vi "mrq_move.vi"(0 "ax":i32, 1 "VISA资源名称":refnum<visa-resource-name>, 2 "page":i32, 3 "t":sgl=1.0, 4 "endV":sgl, 5 "angle":sgl=360.0, 8 "错误输入（无错误）":errorcluster) -> (6 "VISA资源名称输出":refnum<visa-resource-name>, 7 "错误输出":errorcluster)   [LabVIEW 2017]
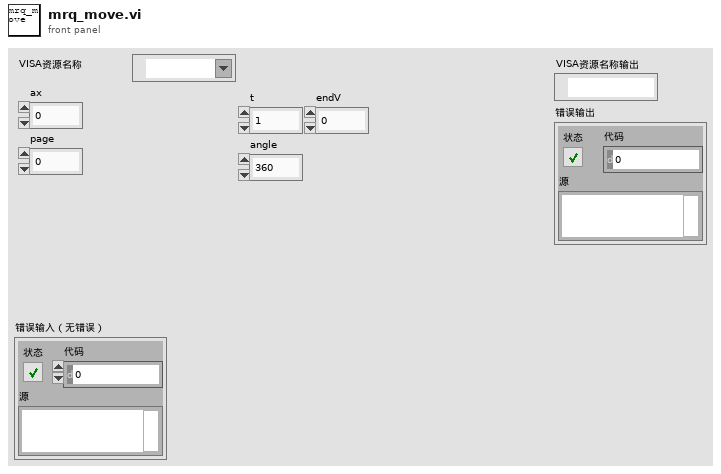
[diagram p1: front panel]
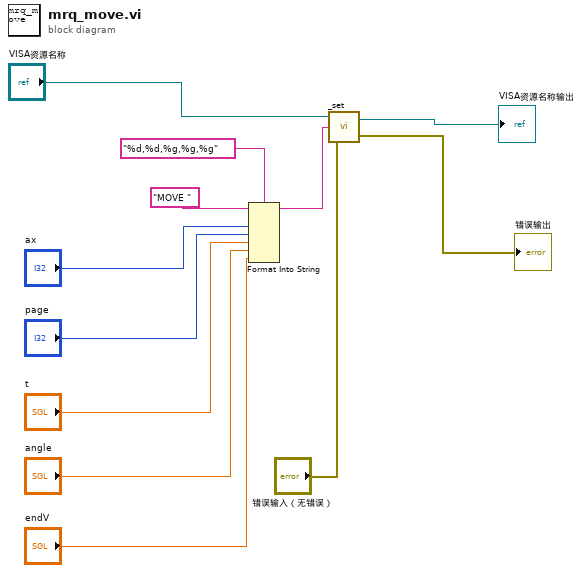
[diagram p0: block diagram]
diagram:
  n1 = Format Into String(format string="%d,%d,%g,%g,%g" ("格式字符串"), initial string="MOVE " ("初始字符串"), "ax", "page", "t", "angle", "endV") -> (resulting string=w11:string)  [unwired: 1 in, 1 out]
  n2 = call "_set.vi"("错误输入（无错误）"="错误输入（无错误）", "写入缓冲区"=w11, "VISA资源名称输出 2"="VISA资源名称") -> ("错误输出"=→"错误输出":errorcluster, "VISA资源名称输出"=→"VISA资源名称输出":refnum<visa-resource-name>)
